vi "Post Message.vi"(8 "error in":errorcluster, 9 "message":string, 11 "Web App Handle In":T1) -> (0 "error out":errorcluster={"status"=FALSE, "code"=5002, "source"=""}, 2 "response":string, 3 "Web App Handle Out":T1)   [LabVIEW 2013, in "Web Messaging API.lvlib"]
doc: "Posts a message to the Web Messaging service, more information can be found at https://myrio.niwsc.com"
uses:
  Web Messaging API.lvlib
  Web Messaging Handle.ctl
  <vilib>/Utility/error.llb/DialogType.ctl
  <vilib>/httpClient/POSTBuffer.vi
  <vilib>/httpClient/LabVIEWHTTPClient.lvlib
panel:
  in  "Message Object":T2={"type"="labview_message", "body"={"und"=[{"value"=" "}]}}
  out "JSON Object":string
  out "headers":string
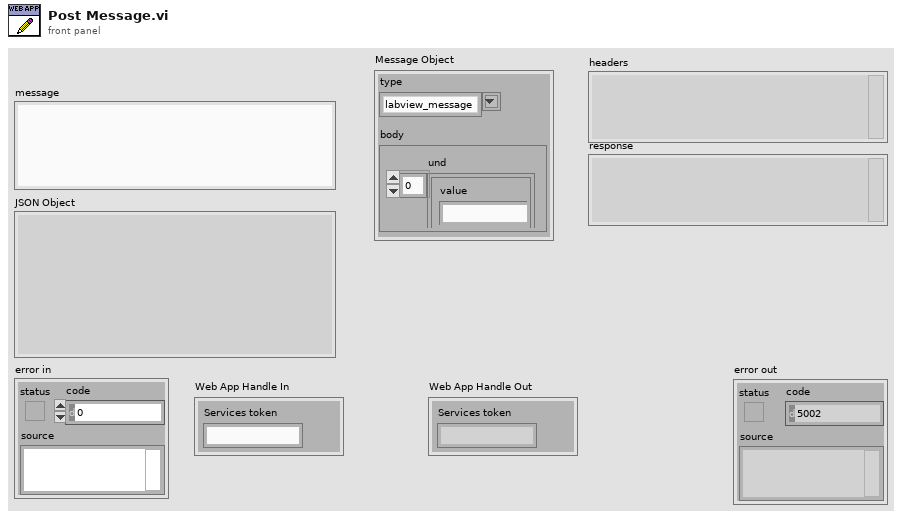
[diagram p1: front panel]
types:
  T1 = typedef "Web Messaging API.lvlib/Web Messaging Handle.ctl" = cluster{"Services token":string}
  T2 = cluster{"type":string, "body":cluster{"und":cluster{"value":string}[]}}
  T3 = typedef "DialogType.ctl" = u16
  T4 = typedef "LabVIEWHTTPClient.lvlib/ClientHandle.ctl" = refnum<k1>
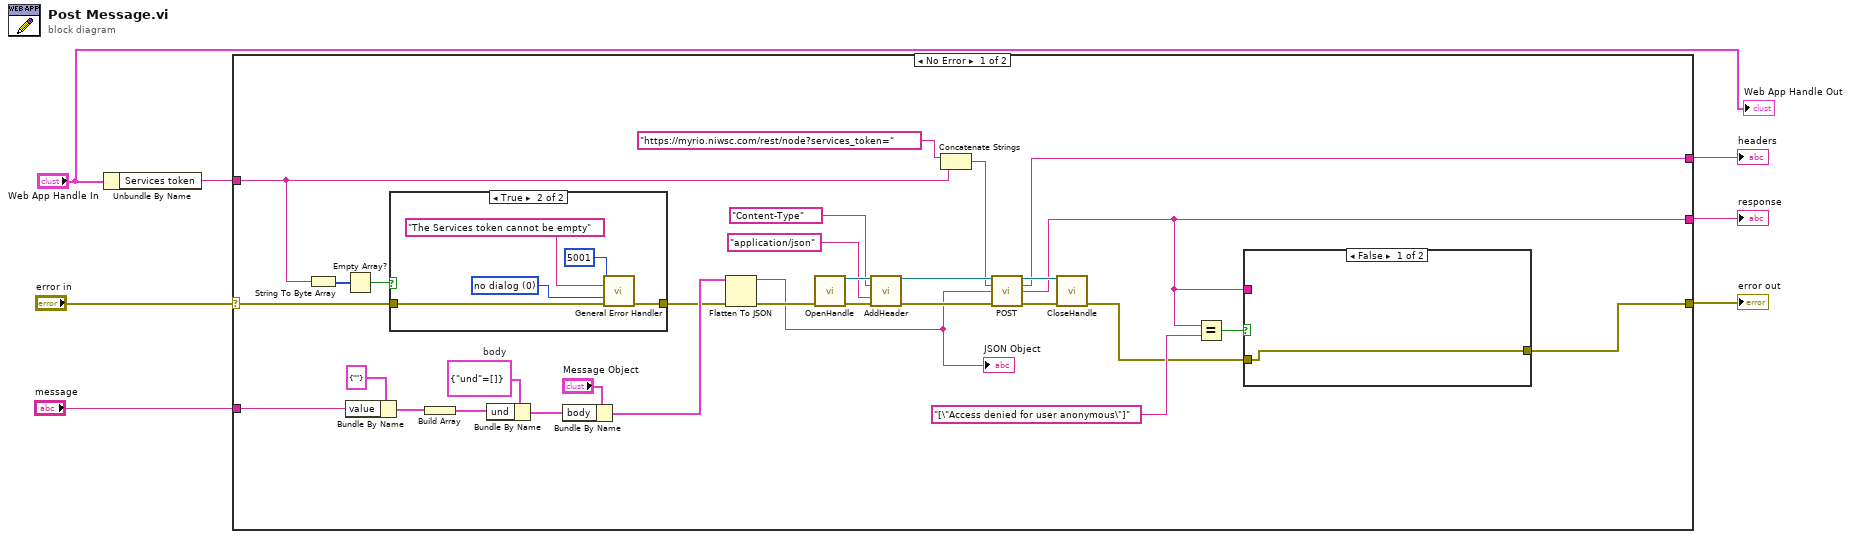
[diagram p0: block diagram]
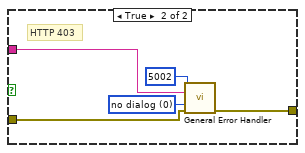
[diagram p2: hidden frame]
diagram:
  n1 = Unbundle By Name("Web App Handle In") -> ("Services token"=w2:string)
  n2 = case shown="No Error" "error in" {
    selector: "error in" -> [w16 w51]
    tunnel: w2 -> [w17 _]
    tunnel: [w8 w51] -> w7
    tunnel: [w28 _] -> w6
    tunnel: [w11 _] -> w5
    tunnel: "message" -> [w20 _]
    frame No Error {
      w25 = cluster{"und":cluster{"value":string}[]} {"und"=[]}  # body
      n3 = String To Byte Array(string=w17) -> (unsigned byte array=w18:u8[])
      n4 = Empty Array?(array=w18) -> (empty?=w19:bool)
      n5 = Bundle By Name(cluster=cluster{"value":string} {"value"=""} ("Cluster"), "value"=w20) -> (w22:cluster{"value":string})
      n6 = case shown="True" w19 {
        tunnel: w16 -> [w45 w48]
        tunnel: [w45 w47] -> w14
        frame False {
        }
        frame True {
          w49 = T3 0 items=["no dialog", "OK message", "continue or stop message", "OK message + warnings", "continue/stop + warnings"] ("type of dialog (OK msg:1)")
          n7 = call <vilib>:"General Error Handler.vi"("[error code] (0)"=5001, "[error source] (\" \")"="The Services token cannot be empty" ("[error source] (\" \")"), "type of dialog (OK msg:1)"=w49, "error in (no error)"=w48) -> ("error out"=w47:errorcluster)  [unwired: 7 in, 4 out]
        }
      }
      n8 = Build Array(w22) -> (w24:cluster{"value":string}[])
      n9 = Bundle By Name(cluster=w25, "und"=w24) -> (w21:cluster{"und":cluster{"value":string}[]})
      n10 = Bundle By Name(cluster="Message Object", "body"=w21) -> (w26:T2)
      n11 = Flatten To JSON(anything=w26, error in (no error)=w14) -> (JSON string=w13:string, 11:w15:errorcluster)  [unwired: 1 in]
      "JSON Object" <- w13
      n12 = call <vilib>:"OpenHandle.vi"("error in (no error)"=w15) -> ("client handle out"=w36:T4, "error out"=w35:errorcluster)  [unwired: 13 in]
      n13 = call <vilib>:"AddHeader.vi"("client handle"=w36, "header"="Content-Type", "value"="application/json", "error in (no error)"=w35) -> ("client handle out"=w31:T4, "error out"=w32:errorcluster)  [unwired: 10 in]
      n14 = Concatenate Strings("https://myrio.niwsc.com/rest/node?services_token=" ("value"), w17) -> (w29:string)
      n15 = call-poly <vilib>:"POST.vi"("client handle"=w31, "url"=w29, "buffer"=w13, "error in (no error)"=w32) -> ("client handle out"=w37:T4, "headers"=w28:string, "body"=w11:string, "error out"=w38:errorcluster)  [unwired: 8 in]
      n16 = call <vilib>:"CloseHandle.vi"("client handle"=w37, "error in (no error)"=w38) -> ("error out"=w9:errorcluster)  [unwired: 13 in]
      n17 = Equal?(x=w11, y="[\"Access denied for user anonymous\"]") -> (x = y?=w12:bool)
      n18 = case shown="False" w12 {
        tunnel: [w39 w43] -> w8
        tunnel: w9 -> [w39 w41]
        tunnel: w11 -> [_ w40]
        frame False {
        }
        frame True {
          w44 = T3 0 items=["no dialog", "OK message", "continue or stop message", "OK message + warnings", "continue/stop + warnings"] ("type of dialog (OK msg:1)")
          # "HTTP 403"
          n19 = call <vilib>:"General Error Handler.vi"("[error code] (0)"=5002, "[error source] (\" \")"=w40, "type of dialog (OK msg:1)"=w44, "error in (no error)"=w41) -> ("error out"=w43:errorcluster)  [unwired: 7 in, 4 out]
        }
      }
    }
    frame Error {
    }
  }
  "error out" <- w7
  "headers" <- w6
  "response" <- w5
  "Web App Handle Out" <- "Web App Handle In"
